vi "encodeMessage.vi"(8 "error in (no error)":errorcluster, 10 "Data in":refnum<class>, 11 "NetworkClient in":refnum<class "NetworkServer.lvclass">) -> (0 "error out":errorcluster, 2 "messageString":string, 3 "NetworkClient out":refnum<class "NetworkServer.lvclass">)   [LabVIEW 2011, in "Hardware.lvlib" / "HWControllers.lvlib" / "NetworkServer.lvclass"]
uses:
  NetworkServer.lvclass
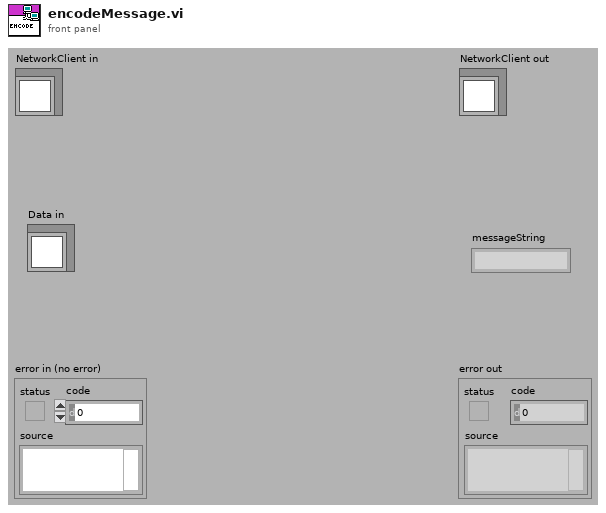
[diagram p1: front panel]
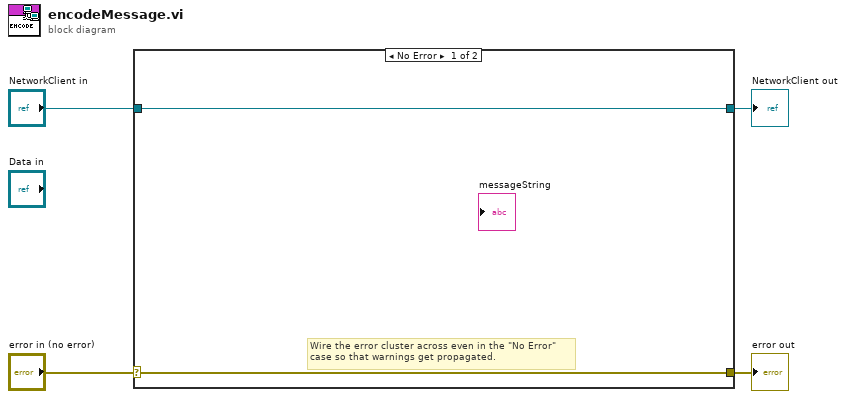
[diagram p0: block diagram]
diagram:
  n1 = case shown="No Error" "error in (no error)" {
    selector: "error in (no error)" -> [w5 w8]
    tunnel: [w5 w8] -> w3
    tunnel: [w6 w7] -> w1
    tunnel: "NetworkClient in" -> [w6 w7]
    frame No Error {
      # "Wire the error cluster across even in the \"No Error\"\ncase so that warnings get propagated."
    }
    frame Error {
    }
  }
  "error out" <- w3
  "NetworkClient out" <- w1
